vi "poly_data_queue_I16.vi"(5 "skip? (F)":bool, 6 "initial queue element (-1)":i16=-1, 7 "initialize":bool, 8 "error in":errorcluster caption="Error in (no error)", 9 "queue length (100)":i32=100, 10 "input data point":i16) -> (0 "error out":errorcluster, 1 "eliminated element":i16, 2 "queue":i16[](array[numeric]), 4 "current length":i32)   [LabVIEW 2015]
uses:
  poly_average_tools_eco_plus.vi
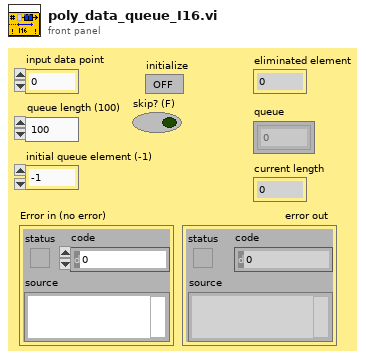
[diagram p1: front panel]
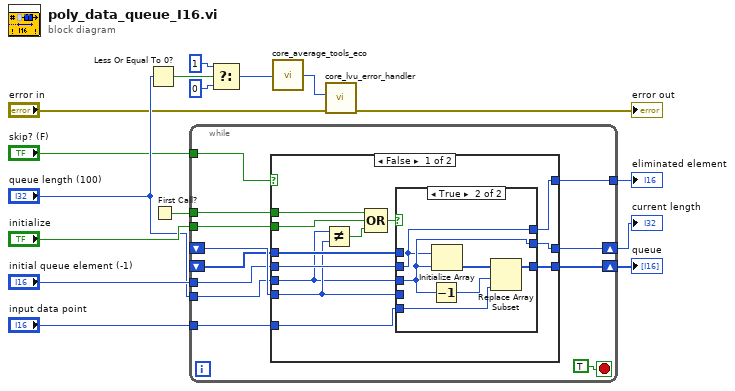
[diagram p0: block diagram]
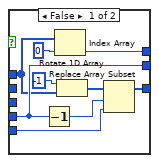
[diagram p2: hidden frame]
diagram:
  n1 = Less Or Equal To 0?(x="queue length (100)") -> (x <= 0?=w8:bool)
  n2 = First Call?() -> (First Call?: T/F=w9:bool)
  n3 = while {
    tunnel: w9 -> [w23]
    shift-left: _ -> [w26]
    shift-right: [w27] -> w15
    shift-left: _ -> [w25]
    shift-right: [w28] -> w16
    tunnel: "initialize" -> [w22]
    tunnel: "input data point" -> [w21]
    tunnel: "initial queue element (-1)" -> [w20]
    tunnel: "queue length (100)" -> [w19]
    tunnel: [w18] -> w11
    tunnel: "skip? (F)" -> [w17]
    stop <- TRUE stop-if-true
    n4 = case shown="False" w17 {
      tunnel: [w40 w58] -> w28
      tunnel: [w39 w57] -> w27
      tunnel: w26 -> [w30 w57]
      tunnel: w25 -> [w38 w58]
      tunnel: w23 -> [w33 _]
      tunnel: w22 -> [w32 _]
      tunnel: w21 -> [w37 w56]
      tunnel: w20 -> [w36 _]
      tunnel: w19 -> [w29 _]
      tunnel: [w35 w56] -> w18
      frame False {
        n5 = Not Equal?(x=w29, y=w30) -> (x != y?=w34:bool)
        n6 = Compound Arithmetic op=OR(w33, w32, w34) -> (w31:bool)
        n7 = case shown="True" w31 {
          tunnel: [w46 w51] -> w40
          tunnel: [w47 w54] -> w39
          tunnel: w30 -> [w47 _]
          tunnel: w38 -> [w43 _]
          tunnel: w37 -> [w48 w52]
          tunnel: w36 -> [_ w50]
          tunnel: w29 -> [_ w54]
          tunnel: [w41 w50] -> w35
          frame False {
            n8 = Decrement(x=w47) -> (x-1=w45:i32)
            n9 = Index Array(array=w43, index=0 ("Index")) -> (element=w41:i16)
            n10 = Rotate 1D Array(1:w43, 2:i16 -1 ("n")) -> (0:w44:i16[])
            n11 = Replace Array Subset(array=w44, new element=w48, index=w45) -> (w46:i16[])
          }
          frame True {
            n12 = Decrement(x=w54) -> (x-1=w55:i32)
            n13 = Initialize Array(w50, w54) -> (w53:i16[])
            n14 = Replace Array Subset(array=w53, new element=w52, index=w55) -> (w51:i16[])
          }
        }
      }
      frame True {
      }
    }
  }
  "queue" <- w16
  "current length" <- w15
  "eliminated element" <- w11
  n15 = Select(t=1, s=w8, f=0) -> (s? t:f=w2:i32)
  n16 = call-poly "core_average_tools_eco.vi"("code (w/out eco)"=w2) -> ("code (+ eco)"=w1:i32)  [unwired: 4 in]
  n17 = call "core_lvu_error_handler.vi"("error in (no error)"="error in", "code (0 = no error)"=w1) -> ("error out"=→"error out":errorcluster)  [unwired: 8 in, 1 out]
